vi "initialise.vi"(8 "error in (no error)":errorcluster, 10 "attribute class to load":T1, 11 "ClassA in":refnum<class "ClassA.lvclass">) -> (0 "error out":errorcluster, 3 "ClassA out":refnum<class "ClassA.lvclass">)   [LabVIEW 2010, in "ClassA.lvclass"]
uses:
  ClassA.lvclass
  attribute_class_enum.ctl
  ClassB/ClassB.lvclass
  ClassA.lvclass/ClassA.ctl
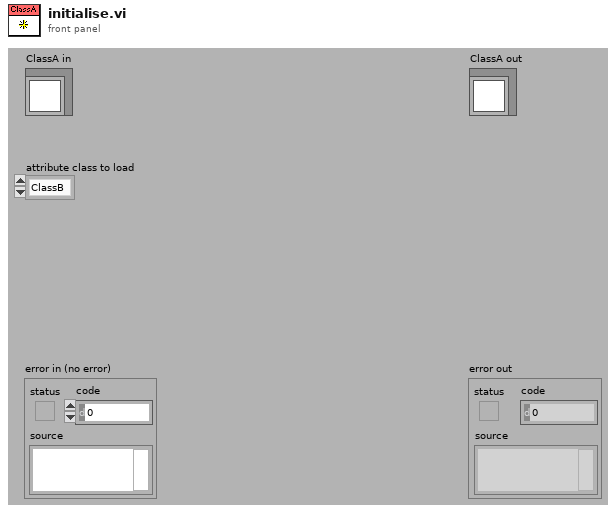
[diagram p1: front panel]
types:
  T1 = typedef "ClassA.lvclass/attribute_class_enum.ctl" = enum16{"ClassB", "ClassC"}
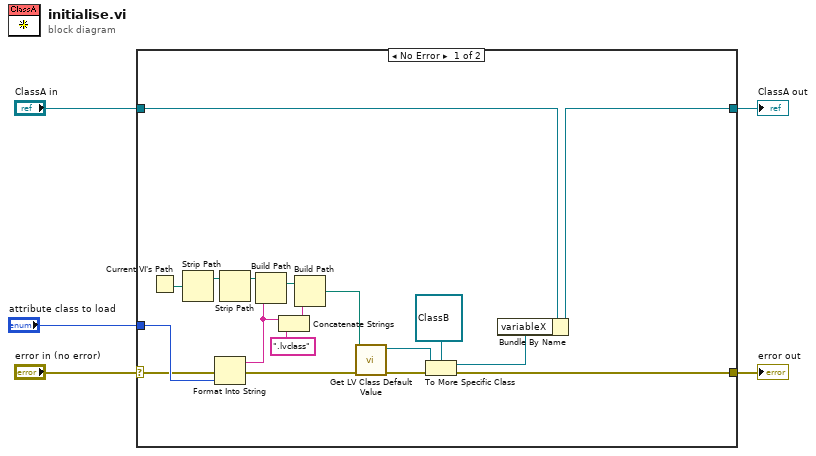
[diagram p0: block diagram]
diagram:
  n1 = case shown="No Error" "error in (no error)" {
    selector: "error in (no error)" -> [w12 w25]
    tunnel: [w20 w25] -> w4
    tunnel: [w17 w24] -> w2
    tunnel: "ClassA in" -> [w18 w24]
    tunnel: "attribute class to load" -> [w13 _]
    frame No Error {
      n2 = Current VI's Path() -> (path=w16:path)
      n3 = Strip Path(path=w16) -> (stripped path=w15:path)  [unwired: 1 out]
      n4 = Format Into String(error in=w12, w13) -> (resulting string=w10:string, error out=w11:errorcluster)  [unwired: 2 in]
      n5 = Strip Path(path=w15) -> (stripped path=w14:path)  [unwired: 1 out]
      n6 = Build Path(base path=w14, name or relative path=w10) -> (appended path=w9:path)
      n7 = Concatenate Strings(w10, ".lvclass" ("string")) -> (w7:string)
      n8 = Build Path(base path=w9, name or relative path=w7) -> (appended path=w6:path)
      n9 = call <vilib>:"Get LV Class Default Value.vi"("error in (no error)"=w11, "class path"=w6) -> ("error out"=w21:errorcluster, "object"=w22:refnum<class>)  [unwired: 8 in]
      n10 = To More Specific Class(target class=refnum<class "ClassB.lvclass"> refnum ("ClassB.lvclass"), reference=w22, error in=w21) -> (specific class reference=w19:refnum<class "ClassB.lvclass">, error out=w20:errorcluster)
      n11 = Bundle By Name(cluster=w18, "variableX"=w19) -> (w17:refnum<class "ClassA.lvclass">)
    }
    frame Error {
    }
  }
  "error out" <- w4
  "ClassA out" <- w2
